vi "RelaysAction_String.vi"(11 "Actions":string) -> (3 "array":T1[](array[typedef]) items=["Open Relay"=20, "Close Relay"=21])   [LabVIEW 2015]
doc: "20- Open relay\n21- Close relay"
uses:
  <instrlib>/niSwitch/niSwitch.llb/niSwitch Relay Action.ctl
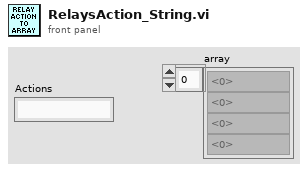
[diagram p1: front panel]
types:
  T1 = typedef "niSwitch Relay Action.ctl" = i32
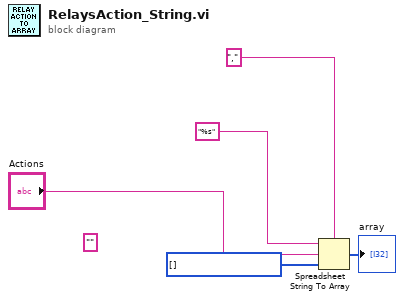
[diagram p0: block diagram]
diagram:
  (unwired) "" ("delimiter (Tab)")
  w3 = T1[] [] items=["Open Relay"=20, "Close Relay"=21]
  n1 = Spreadsheet String To Array(delimiter (Tab)=",", format string="%s", spreadsheet string="Actions", array type (2D Dbl)=w3) -> (array=→"array":T1[])
